vi "Encode ACW Parameters.vi"(8 "ADD Parameters (in)":string, 9 "Scanner Settings In":T2={"Scan1"=1, "Scan2"=1, "Scan3"=1, "Scan4"=1, "Scan5"=1, "Scan6"=1, "Scan7"=1, "Scan8"=1, "Scan9"=1, "Scan10"=1, "Scan11"=1, "Scan12"=1, "Scan13"=1, "Scan14"=1, "Scan15"=1, "Scan16"=1} {"Scan16" scale=0.0..2.0; "Scan15" scale=0.0..2.0; "Scan14" scale=0.0..2.0; "Scan13" scale=0.0..2.0; "Scan12" scale=0.0..2.0; "Scan11" scale=0.0..2.0; "Scan10" scale=0.0..2.0; "Scan9" scale=0.0..2.0; "Scan8" scale=0.0..2.0; "Scan7" scale=0.0..2.0; "Scan6" scale=0.0..2.0; "Scan5" scale=0.0..2.0; "Scan4" scale=0.0..2.0; "Scan3" min=0 max=2 scale=0.0..2.0; "Scan2" min=0 max=2 scale=0.0..2.0; "Scan1" min=0 max=2 scale=0.0..2.0}, 10 "Internal Scanner Exists?":bool, 11 "ACW Test Parameters (in)":T1={"Voltage (0~5.0 KV)"=1.0, "High Limit(0.0~20.00 mA)"=0.0, "Low Limit(0~10.00 mA)"=0.0, "Ramp Up Time (0.1~999.9 seconds)"=0.4, "Dwell Time (0, 0.3~999.9 seconds)"=1.0, "Ramp Down Time (0~999.9 seconds)"=0.0, "Arc Sense (1~9)"=5, "Arc Detect (F: Off)"=FALSE, "Frequency (50/60 Hz)"=50} {"Ramp Down Time (0~999.9 seconds)" format="%.1f"; "Arc Sense (1~9)" format="%.3f"; "Dwell Time (0, 0.3~999.9 seconds)" format="%.1f"; "Ramp Up Time (0.1~999.9 seconds)" format="%.1f"; "Low Limit(0~10.00 mA)" format="%.1f"; "High Limit(0.0~20.00 mA)" format="%.1f"; "Voltage (0~5.0 KV)" format="%.1f"}) -> (1 "ACW Test Parameters (out)":T1={"Voltage (0~5.0 KV)"=1.0, "High Limit(0.0~20.00 mA)"=0.0, "Low Limit(0~10.00 mA)"=0.0, "Ramp Up Time (0.1~999.9 seconds)"=0.4, "Dwell Time (0, 0.3~999.9 seconds)"=1.0, "Ramp Down Time (0~999.9 seconds)"=0.0, "Arc Sense (1~9)"=5, "Arc Detect (F: Off)"=FALSE, "Frequency (50/60 Hz)"=50} {"Ramp Down Time (0~999.9 seconds)" format="%.1f"; "Arc Sense (1~9)" format="%.3f"; "Dwell Time (0, 0.3~999.9 seconds)" format="%.1f"; "Ramp Up Time (0.1~999.9 seconds)" format="%.1f"; "Low Limit(0~10.00 mA)" format="%.1f"; "High Limit(0.0~20.00 mA)" format="%.1f"; "Voltage (0~5.0 KV)" format="%.1f"}, 2 "Scanner Settings Out":T2={"Scan1"=1, "Scan2"=1, "Scan3"=1, "Scan4"=1, "Scan5"=1, "Scan6"=1, "Scan7"=1, "Scan8"=1, "Scan9"=1, "Scan10"=1, "Scan11"=1, "Scan12"=1, "Scan13"=1, "Scan14"=1, "Scan15"=1, "Scan16"=1} {"Scan16" scale=0.0..2.0; "Scan15" scale=0.0..2.0; "Scan14" scale=0.0..2.0; "Scan13" scale=0.0..2.0; "Scan12" scale=0.0..2.0; "Scan11" scale=0.0..2.0; "Scan10" scale=0.0..2.0; "Scan9" scale=0.0..2.0; "Scan8" scale=0.0..2.0; "Scan7" scale=0.0..2.0; "Scan6" scale=0.0..2.0; "Scan5" scale=0.0..2.0; "Scan4" scale=0.0..2.0; "Scan3" min=0 max=2 scale=0.0..2.0; "Scan2" min=0 max=2 scale=0.0..2.0; "Scan1" min=0 max=2 scale=0.0..2.0}, 3 "Add Parameters":string)   [LabVIEW 2016, in "EEC EST 300.lvlib"]
uses:
  <instrlib>/eec EST 300/eec EST 300.lvlib
  <instrlib>/eec EST 300/Public/Configure/Steps/Low Level/Scanner Settings.ctl
  <instrlib>/eec EST 300/Public/Configure/Steps/Low Level/ACW Test Parameters.ctl
panel:
  out "output 7":string
  # "On\nOff"
  # "On\nOff"
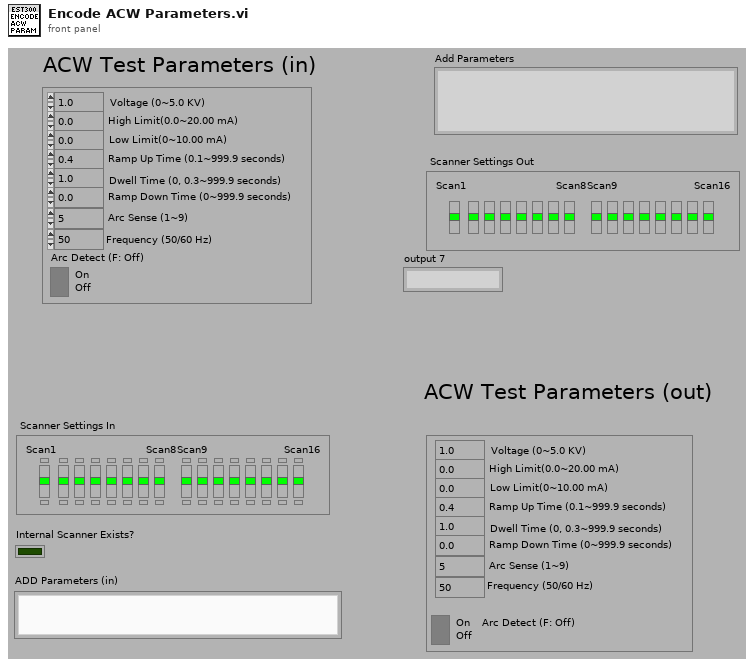
[diagram p1: front panel]
types:
  T1 = typedef "EEC EST 300.lvlib/ACW Test Parameters.ctl" = cluster{"Voltage (0~5.0 KV)":dbl, "High Limit(0.0~20.00 mA)":dbl, "Low Limit(0~10.00 mA)":dbl, "Ramp Up Time (0.1~999.9 seconds)":dbl, "Dwell Time (0, 0.3~999.9 seconds)":dbl, "Ramp Down Time (0~999.9 seconds)":dbl, "Arc Sense (1~9)":i32, "Arc Detect (F: Off)":bool, "Frequency (50/60 Hz)":i32}
  T2 = typedef "eec EST 300.lvlib/Scanner Settings.ctl" = cluster{"Scan1":i32, "Scan2":i32, "Scan3":i32, "Scan4":i32, "Scan5":i32, "Scan6":i32, "Scan7":i32, "Scan8":i32, "Scan9":i32, "Scan10":i32, "Scan11":i32, "Scan12":i32, "Scan13":i32, "Scan14":i32, "Scan15":i32, "Scan16":i32}
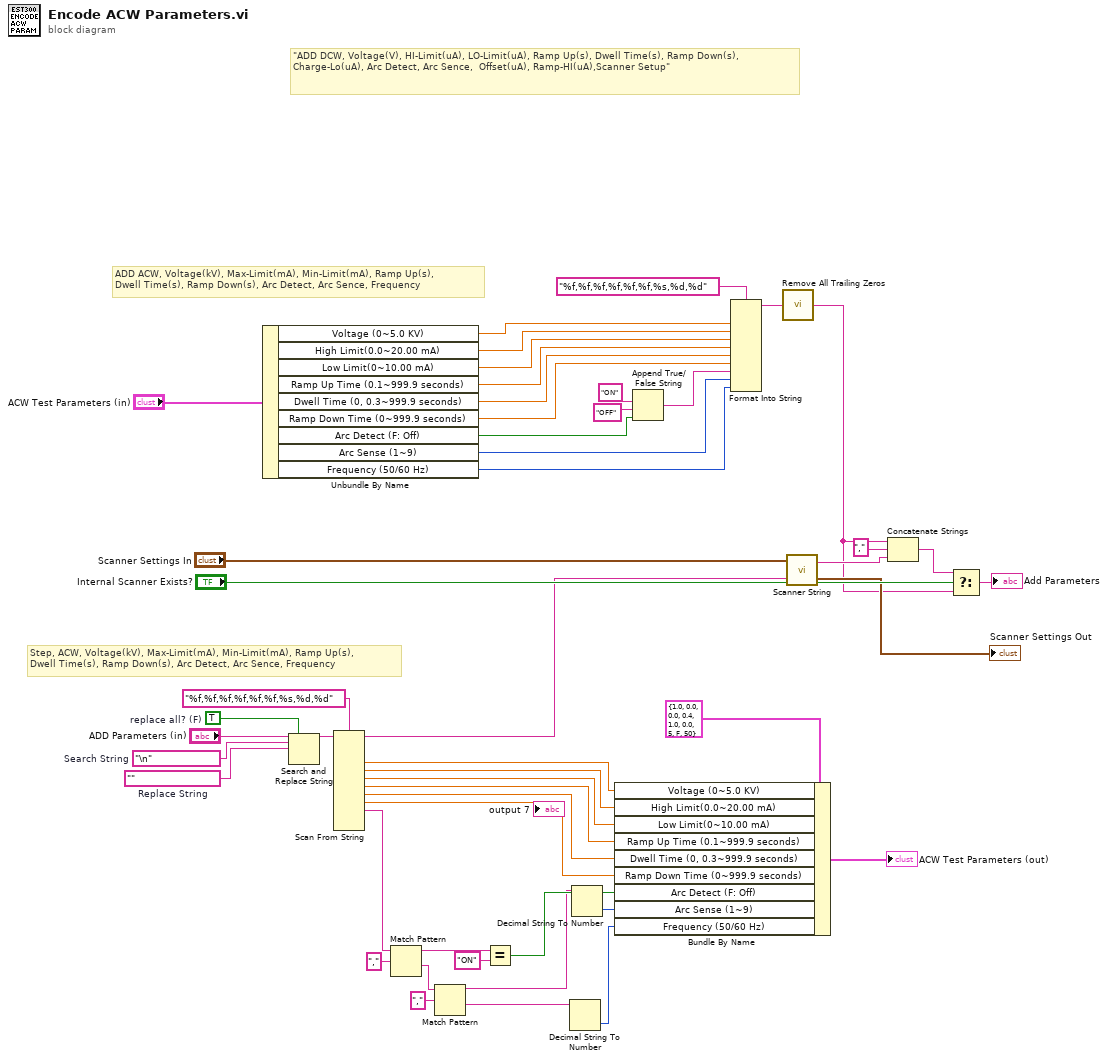
[diagram p0: block diagram]
diagram:
  w38 = TRUE  # replace all? (F)
  w39 = ""  # Replace String
  w40 = "\n"  # Search String
  # "Step, ACW, Voltage(kV), Max-Limit(mA), Min-Limit(mA), Ramp Up(s), \nDwell Time(s), Ramp Down(s), Arc Detect, Arc Sence, Frequency"
  # "ADD ACW, Voltage(kV), Max-Limit(mA), Min-Limit(mA), Ramp Up(s), \nDwell Time(s), Ramp Down(s), Arc Detect, Arc Sence, Frequency"
  # "\"ADD DCW, Voltage(V), HI-Limit(uA), LO-Limit(uA), Ramp Up(s), Dwell Time(s), Ramp Down(s), \nCharge-Lo(uA), Arc Detect, Arc Sence,  Offset(uA), Ramp-HI(uA),Scanner Setup\""
  n1 = Unbundle By Name("ACW Test Parameters (in)") -> ("Voltage (0~5.0 KV)"=w49:dbl, "High Limit(0.0~20.00 mA)"=w33:dbl, "Low Limit(0~10.00 mA)"=w48:dbl, "Ramp Up Time (0.1~999.9 seconds)"=w47:dbl, "Dwell Time (0, 0.3~999.9 seconds)"=w46:dbl, "Ramp Down Time (0~999.9 seconds)"=w45:dbl, "Arc Detect (F: Off)"=w32:bool, "Arc Sense (1~9)"=w30:i32, "Frequency (50/60 Hz)"=w29:i32)
  n2 = Search and Replace String(replace all?=w38, input string="ADD Parameters (in)", search string=w40, replace string=w39) -> (result string=w36:string)  [unwired: 4 in, 3 out]
  n3 = Scan From String(format string="%f,%f,%f,%f,%f,%f,%s,%d,%d" ("Format String"), input string=w36) -> (remaining string=w24:string, output 1=w17:dbl, output 2=w14:dbl, output 3=w15:dbl, output 4=w16:dbl, output 5=w13:dbl, output 6=w12:dbl, output 7=w11:string)  [unwired: 13 in, 2 out]
  n4 = Match Pattern(string=w11, regular expression=",") -> (before substring=w7:string, after substring=w5:string)  [unwired: 1 in, 2 out]
  n5 = Match Pattern(string=w5, regular expression=",") -> (before substring=w4:string, after substring=w1:string)  [unwired: 1 in, 2 out]
  n6 = Equal?(x=w7, y="ON") -> (x = y?=w8:bool)
  n7 = Decimal String To Number(string=w1) -> (number=w2:i32)  [unwired: 2 in, 1 out]
  n8 = Decimal String To Number(string=w4) -> (number=w3:i32)  [unwired: 2 in, 1 out]
  n9 = Bundle By Name(cluster=T1 {"Voltage (0~5.0 KV)"=1.0, "High Limit(0.0~20.00 mA)"=0.0, "Low Limit(0~10.00 mA)"=0.0, "Ramp Up Time (0.1~999.9 seconds)"=0.4, "Dwell Time (0, 0.3~999.9 seconds)"=1.0, "Ramp Down Time (0~999.9 seconds)"=0.0, "Arc Sense (1~9)"=5, "Arc Detect (F: Off)"=FALSE, "Frequency (50/60 Hz)"=50} ("ACW Test Parameters (out) 2"), "Voltage (0~5.0 KV)"=w17, "High Limit(0.0~20.00 mA)"=w14, "Low Limit(0~10.00 mA)"=w15, "Ramp Up Time (0.1~999.9 seconds)"=w16, "Dwell Time (0, 0.3~999.9 seconds)"=w13, "Ramp Down Time (0~999.9 seconds)"=w12, "Arc Detect (F: Off)"=w8, "Arc Sense (1~9)"=w3, "Frequency (50/60 Hz)"=w2) -> (→"ACW Test Parameters (out)":T1)
  n10 = Append True/False String(1:w32, 2:"OFF" ("false string"), 3:"ON" ("true string")) -> (0:w31:string)  [unwired: 1 in]
  n11 = Format Into String(format string="%f,%f,%f,%f,%f,%f,%s,%d,%d" ("Format String"), w49, w33, w48, w47, w46, w45, w31, w30, w29) -> (resulting string=w23:string)  [unwired: 2 in, 1 out]
  n12 = call <instrlib>:"Remove All Trailing Zeros.vi"("String in"=w23) -> ("String out"=w22:string)
  n13 = call <instrlib>:"Scanner String.vi"("Scanner String (in)"=w24, "Scanner Settings in"="Scanner Settings In") -> ("Scanner Settings out"=→"Scanner Settings Out":T2, "Scanner String (out)"=w25:string)
  n14 = Concatenate Strings(w22, "," ("Substring"), w25) -> (w41:string)
  n15 = Select(t=w41, s="Internal Scanner Exists?", f=w22) -> (s? t:f=→"Add Parameters":string)
